vi "DDOdom_Abs_TrajCreation.vi"(8 "Destination Waypoint":T7={"TRANSLATION"={"X"=0.0, "Y"=0.0}, "ROTATION"={"VALUE"=0.0, "COS"=1.0, "SIN"=0.0}, "SCALAR"=-45.0} {"SCALAR" format="%14.3f"; "ROTATION"."SIN" format="%13.4f"; "ROTATION"."COS" format="%13.4f"; "ROTATION"."VALUE" format="%13.4f"; "TRANSLATION"."Y" format="%14.3f"; "TRANSLATION"."X" format="%14.3f"}, 9 "Initial Waypoint":T7={"TRANSLATION"={"X"=0.0, "Y"=0.0}, "ROTATION"={"VALUE"=0.0, "COS"=1.0, "SIN"=0.0}, "SCALAR"=-45.0} {"SCALAR" format="%14.3f"; "ROTATION"."SIN" format="%13.4f"; "ROTATION"."COS" format="%13.4f"; "ROTATION"."VALUE" format="%13.4f"; "TRANSLATION"."Y" format="%14.3f"; "TRANSLATION"."X" format="%14.3f"}, 10 "Effective Track Width Ft":dbl=5.83 format="%17.3f", 11 "Max Velocity Ft/Sec":dbl=5.55 format="%17.3f") -> (0 "Trajectory  creation error":errorcluster, 1 "Absolute Trajectory":T1 {"States"."POSE"."ROTATION"."SIN" format="%13.4f"; "States"."POSE"."ROTATION"."COS" format="%13.4f"; "States"."POSE"."ROTATION"."VALUE" format="%13.4f"; "States"."POSE"."TRANSLATION"."Y" format="%14.3f"; "States"."POSE"."TRANSLATION"."X" format="%14.3f"; "TotalTImeSecs" format="%20.3f"}, 2 "Trajectory Items":i32, 3 "TotalTImeSecs":dbl)   [LabVIEW 2019]
uses:
  <vilib>/Rock Robotics/WPI/ThirdParty/JAS_Junk/TrajLib/TypeDef/WEIGHTED_WAYPOINT.ctl
  <vilib>/Rock Robotics/WPI/ThirdParty/JAS_Junk/TrajLib/TypeDef/TRANSLATION2D.ctl
  <vilib>/Rock Robotics/WPI/ThirdParty/JAS_Junk/TrajLib/TypeDef/ROTATION2D.ctl
  <vilib>/Rock Robotics/WPI/ThirdParty/JAS_Junk/TrajLib/Enum/TRAJECTORY_SPLINE_TYPE_ENUM.ctl
  <vilib>/Rock Robotics/WPI/ThirdParty/JAS_Junk/TrajLib/TypeDef/TRAJECTORY.ctl
  <vilib>/Rock Robotics/WPI/ThirdParty/JAS_Junk/TrajLib/TypeDef/TRAJ_STATE.ctl
  <vilib>/Rock Robotics/WPI/ThirdParty/JAS_Junk/TrajLib/TypeDef/POSE2D.ctl
  <vilib>/Rock Robotics/SystemInterfaces/NetworkCommunication/NetComm_UsageReport_report.vi
  <vilib>/Rock Robotics/WPI/ThirdParty/JAS_Junk/TrajLib/DiffDriveKinematicsConstraint_New.vi
  <vilib>/Rock Robotics/WPI/ThirdParty/JAS_Junk/TrajLib/TrajectoryConfig_AddConstraint.vi
  <vilib>/Rock Robotics/WPI/ThirdParty/JAS_Junk/TrajLib/CentripetalAccelConstraint_New.vi
  <vilib>/Rock Robotics/WPI/ThirdParty/JAS_Junk/TrajLib/Globals/Util_LibraryGlobals.vi
  <vilib>/Rock Robotics/WPI/ThirdParty/JAS_Junk/TrajLib/Trajectory_Library.lvlib
panel:
  out "Trajectory":cluster{dbl[], dbl[]}[](graph)
  in  "Spline Type":T6
  in  "Use Diff Drive\nKinematic\nConstraint":bool=TRUE
  in  "Use Centripetal\nAcceleration\nConstaint":bool=TRUE
  out "Track Width_M":dbl=0.66 format="%20.4f"
  out "MaxAcceleration  M/S^2":dbl=1.3 format="%17.4f"
  out "MaxVelocity M/S":dbl=2.0 format="%17.4f"
  out "Max Cent Accel":dbl=1.0 format="%20.4f"
  in  "Max Cent Accel INCHES/SEC^2":dbl=15.0 format="%20.1f"
  in  "MaxAcceleration INCHES/SEC^2":dbl=30.0 format="%17.1f"
  in  "MaxVelocity Fraction":dbl=0.66 format="%17.3f"
  # "This creates an absolute trajectory."
  # "CREATED TRAJECTORY INFORMATION"
  # "TRAJECTORY CONFIGURATION"
  # "real sim robot 20.9 inch"
  # "TRAJECTORY DEFINITION"
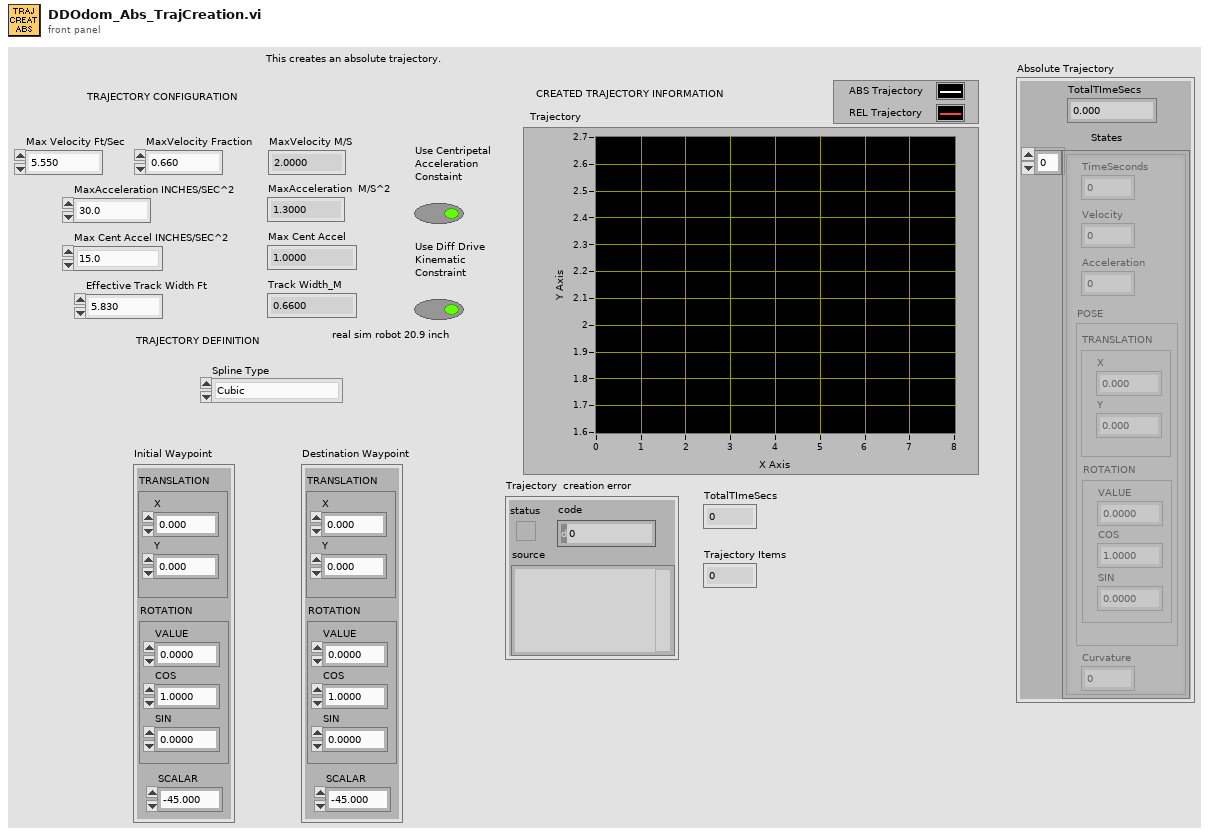
[diagram p1: front panel]
types:
  T1 = typedef "Trajectory_Library.lvlib/TRAJECTORY.ctl" = cluster{"TotalTImeSecs":dbl, "States":T2[]}
  T2 = typedef "Trajectory_Library.lvlib/TRAJ_STATE.ctl" = cluster{"TimeSeconds":dbl, "Velocity":dbl, "Acceleration":dbl, "POSE":T3, "Curvature":dbl}
  T3 = typedef "Trajectory_Library.lvlib/POSE2D.ctl" = cluster{"TRANSLATION":T4, "ROTATION":T5}
  T4 = typedef "Trajectory_Library.lvlib/TRANSLATION2D.ctl" = cluster{"X":dbl, "Y":dbl}
  T5 = typedef "Trajectory_Library.lvlib/ROTATION2D.ctl" = cluster{"VALUE":dbl, "COS":dbl, "SIN":dbl}
  T6 = typedef "Trajectory_Library.lvlib/TRAJECTORY_SPLINE_TYPE_ENUM.ctl" = enum16{"Cubic", "Cubic With Weights", "Quintic", "Quintic With Weights"}
  T7 = typedef "Trajectory_Library.lvlib/WEIGHTED_WAYPOINT.ctl" = cluster{"TRANSLATION":T4, "ROTATION":T5, "SCALAR":dbl}
  T8 = typedef "Trajectory_Library.lvlib/TRAJ_CONFIG.ctl" = cluster{"MaxVelocity":dbl, "Max Acceleration":dbl, "StartVelocity":dbl, "End Velocity":dbl, "Reversed":bool, "Constraints":variant[]}
  T9 = typedef "Trajectory_Library.lvlib/DIFF_DRIVE_KINEMATICS.ctl" = cluster{"TrackWidth_Meters":dbl}
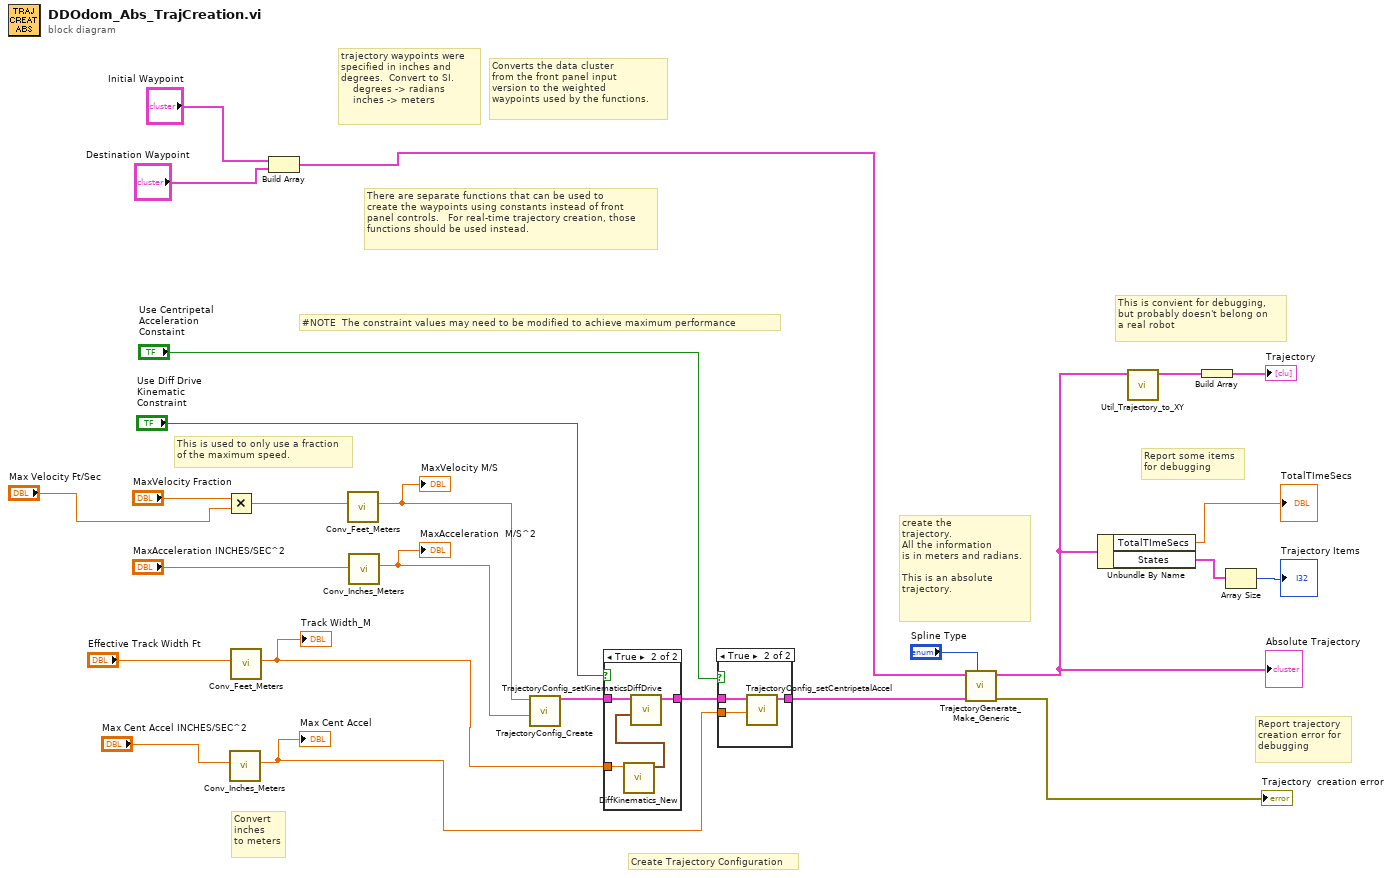
[diagram p0: block diagram]
diagram:
  # "There are separate functions that can be used to \ncreate the waypoints using constants instead of front\npanel controls.   For real-time trajectory creation, those\nfunctions should be used instead."
  # "This is convient for debugging,\nbut probably doesn't belong on\na real robot"
  # "This is used to only use a fraction\nof the maximum speed."
  # "Report trajectory\ncreation error for \ndebugging"
  # "Report some items\nfor debugging"
  # "Converts the data cluster\nfrom the front panel input\nversion to the weighted \nwaypoints used by the functions."
  # "#NOTE  The constraint values may need to be modified to achieve maximum performance"
  # "Convert\ninches\nto meters"
  # "create the\ntrajectory.\nAll the information\nis in meters and radians.\n\nThis is an absolute \ntrajectory."
  # "trajectory waypoints were \nspecified in inches and\ndegrees.  Convert to SI.\n    degrees -> radians\n    inches -> meters"
  # "Create Trajectory Configuration"
  n1 = Multiply(x="MaxVelocity Fraction", y="Max Velocity Ft/Sec") -> (x*y=w11:dbl)
  n2 = call <vilib>:"Conv_Inches_Meters.vi"("INCH"="Max Cent Accel INCHES/SEC^2") -> ("Meters"=w19:dbl)  [unwired: 10 in]
  "Max Cent Accel" <- w19
  n3 = call <vilib>:"Conv_Feet_Meters.vi"("Feet"="Effective Track Width Ft") -> ("Meters"=w20:dbl)  [unwired: 10 in]
  "Track Width_M" <- w20
  n4 = Build Array("Initial Waypoint", "Destination Waypoint") -> (w2:T7[])
  n5 = call <vilib>:"Conv_Feet_Meters.vi"("Feet"=w11) -> ("Meters"=w17:dbl)  [unwired: 10 in]
  "MaxVelocity M/S" <- w17
  n6 = call <vilib>:"Conv_Inches_Meters.vi"("INCH"="MaxAcceleration INCHES/SEC^2") -> ("Meters"=w18:dbl)  [unwired: 10 in]
  "MaxAcceleration  M/S^2" <- w18
  n7 = call <vilib>:"TrajectoryConfig_Create.vi"("MaxAcceleration"=w18, "MaxVelocity"=w17) -> ("TRAJECTORY_CONFIG"=w24:T8)  [unwired: 9 in]
  n8 = case shown="True" "Use Diff Drive\nKinematic\nConstraint" {
    tunnel: w24 -> [w27 w31]
    tunnel: [w27 w30] -> w23
    tunnel: w20 -> [_ w28]
    frame False {
    }
    frame True {
      n9 = call <vilib>:"DiffKinematics_New.vi"("TrackWidth_Meters"=w28) -> ("DIFF_DRIVE_KINEMATICS"=w29:T9)  [unwired: 10 in]
      n10 = call <vilib>:"TrajectoryConfig_setKinematicsDiffDrive.vi"("DIFF_DRIVE_KINEMATICS"=w29, "inTRAJECTORY_CONFIG"=w31) -> ("outTRAJECTORY_CONFIG"=w30:T8)  [unwired: 9 in]
    }
  }
  n11 = case shown="True" "Use Centripetal\nAcceleration\nConstaint" {
    tunnel: w23 -> [w32 w35]
    tunnel: [w32 w34] -> w15
    tunnel: w19 -> [_ w33]
    frame False {
    }
    frame True {
      n12 = call <vilib>:"TrajectoryConfig_setCentripetalAccel.vi"("Max Cent Accel"=w33, "inTRAJECTORY_CONFIG"=w35) -> ("outTRAJECTORY_CONFIG"=w34:T8)  [unwired: 9 in]
    }
  }
  n13 = call <vilib>:"TrajectoryGenerate_Make_Generic.vi"("Spline Type"="Spline Type", "traj_config"=w15, "WeightedWayPoints"=w2) -> ("error out"=→"Trajectory  creation error":errorcluster, "TRAJECTORY"=w3:T1)  [unwired: 7 in]
  "Absolute Trajectory" <- w3
  n14 = Unbundle By Name(w3) -> ("TotalTImeSecs"=→"TotalTImeSecs":dbl, "States"=w13:T2[])
  n15 = call <vilib>:"Util_Trajectory_to_XY.vi"("TRAJECTORY"=w3) -> ("outArrayXY"=w8:cluster{dbl[], dbl[]})  [unwired: 10 in]
  n16 = Build Array(w8) -> (→"Trajectory":cluster{dbl[], dbl[]}[])
  n17 = Array Size(array=w13) -> (size(s)=→"Trajectory Items":i32)
